vi "FGV_LoopRunner.vi"(1 "Loop Controller":T1(ring)) -> (0 "Stop Loops":bool)   [LabVIEW 2014]
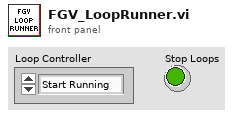
[diagram p1: front panel]
types:
  T1 = enum16{"Start Running", "Stop Running", "Check State"}
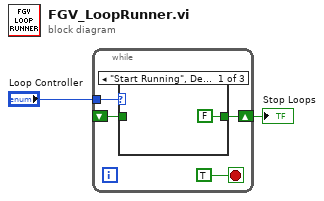
[diagram p0: block diagram]
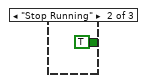
[diagram p2: hidden frame]
diagram:
  n1 = while {
    tunnel: "Loop Controller" -> [w5]
    shift-right: [w4] -> w2
    shift-left: _ -> [w3]
    stop <- TRUE stop-if-true
    n2 = case shown="\"Start Running\", Default" w5 {
      tunnel: [FALSE TRUE w9] -> w4
      tunnel: w3 -> [_ _ w9]
      frame "Start Running", Default {
      }
      frame "Stop Running" {
      }
      frame "Check State" {
      }
    }
  }
  "Stop Loops" <- w2
